vi "VCS Set Max Following Error.vi"(8 "error in (no error)":errorcluster, 9 "maxFollowingError":u32, 11 "axis in":cluster{"keyHandle":u32, "nodeId":u16}={"keyHandle"=0, "nodeId"=1}) -> (0 "error out":errorcluster, 3 "axis out":cluster{"keyHandle":u32, "nodeId":u16}={"keyHandle"=0, "nodeId"=1})   [LabVIEW 2018]
doc: "<B>VCS_SetMaxFollowingError</B> writes the maximal allowed following error parameter."
uses:
  Resources/EposCmd.dll
  Resources/EposCmd64.dll
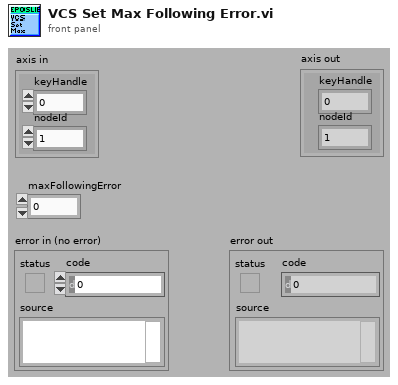
[diagram p1: front panel]
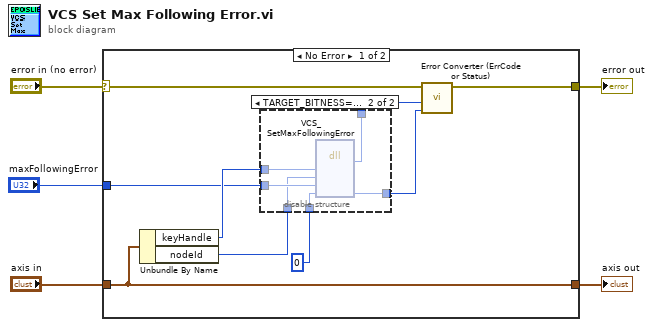
[diagram p0: block diagram]
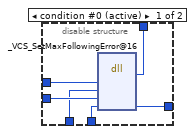
[diagram p2: hidden frame]
diagram:
  n1 = case shown="No Error" "error in (no error)" {
    selector: "error in (no error)" -> [w12 w27]
    tunnel: "axis in" -> [w14 w28]
    tunnel: [w14 w28] -> w4
    tunnel: [w13 w27] -> w3
    tunnel: "maxFollowingError" -> [w7 _]
    frame No Error {
      n2 = Unbundle By Name(w14) -> ("keyHandle"=w10:u32, "nodeId"=w6:u16)
      n3 = disable-structure shown="TARGET_BITNESS==64" {
        disable-tunnel: u32 0 ("pErrorCode") -> [w20 w26]
        disable-tunnel: w10 -> [w19 w25]
        disable-tunnel: [w18 w24] -> w9
        disable-tunnel: [w17 w23] -> w8
        disable-tunnel: w7 -> [w16 w22]
        disable-tunnel: w6 -> [w15 w21]
        frame condition #0 (active) {
          n4 = dll-call lib="C:/Projeto em LabVIEW/EPOS-LabVIEW-Instrument-Driver-En/LabVIEW/maxon EPOS/Resources/EposCmd.*" fn="_VCS_SetMaxFollowingError@16"("KeyHandle"=w19, "NodeId"=w15, "MaxFollowingError"=w16, "pErrorCode"=w20) -> (w18:i32, "pErrorCode"=w17:u32)  [unwired: 6 in, 2 out]
        }
        frame condition #1 {
          n5 = dll-call lib="C:/setup/Resources/EposCmd64.*" fn="VCS_SetMaxFollowingError" ("EposCmd.dll:_VCS_SetMaxFollowingError@16")("KeyHandle"=w25, "NodeId"=w21, "MaxFollowingError"=w22, "pErrorCode"=w26) -> ("Rückgabetyp"=w24:i32, "pErrorCode"=w23:u32)  [unwired: 6 in, 2 out]
        }
      }
      n6 = call "Error Converter (ErrCode or Status).vi"("error code"=w8, "return type"=w9, "error in (no error)"=w12) -> ("error out"=w13:errorcluster)  [unwired: 7 in]
    }
    frame Error {
    }
  }
  "error out" <- w3
  "axis out" <- w4
